vi "niFpgaRegisterEmulationRefIn.vi"(0 "Name":variant, 1 "in timed loop":bool, 7 "Data In":i32, 9 "Write? (F)":bool, 11 "error in (no error)":errorcluster, 12 "Node Link":cluster{"VIRef":refnum<vi>, "UID":i32}) -> (8 "Data Out":i32, 15 "error out":errorcluster)   [LabVIEW 2017]
uses:
  <vilib>/rvi/DataTransferAndStorage/Container/Common/niFpgaContainerMetaDataKey.ctl
  <instcachedir>/0/niFpgaRegisterEmulation_D83EC659CC8640A8A24FC76F9511FEDC.lvgen/niFpgaRegisterEmulation_D83EC659CC8640A8A24FC76F9511FEDC_000.vi
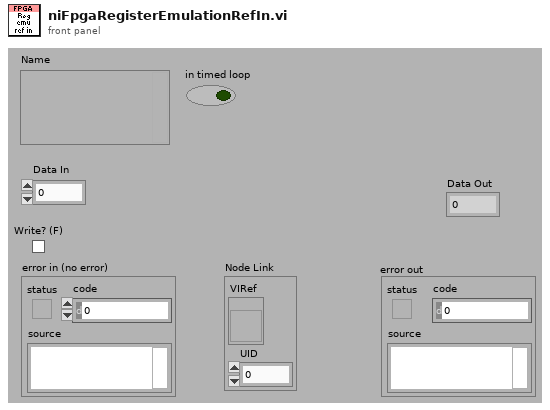
[diagram p1: front panel]
types:
  T1 = typedef "niFpgaContainerMetaDataKey.ctl" = enum16{"FPGA FIFO", "FPGA Memory", "FPGA Register", "FPGA Handshake"}
  T2 = typedef "niFpgaContainerState.ctl" = cluster{"displayName":string, "hardwareName":string, "dataType":T3, "elementTypeDescriptor":variant, "terminalTypeDescriptor":variant, "requestedNumberOfElements":u32, "memoryType":T4, "arbitrationForInterfaceA":T5, "numberOfElementsPerRead":u32, "arbitrationForInterfaceB":T5, "numberOfElementsPerWrite":u32, "VI_Defined":bool, "type":T6, "initializationParameters":T7, "disableOnOverflow/Underflow":bool, "interfaceConfiguration":T8, "controlLogic":T9, "actualNumberOfElements":u32, "dramSelection":string, "dramMaxOustandingRequests":i32, "dramIncludeByteEnables":bool, "dramGrantTime":u32, "fullEmulation":bool, "memoryInMultipleClockDomains":bool, "memoryLatency":T10}
  T3 = typedef "niFpgaDataTypeControl.ctl" = enum32{"Boolean", "I8", "I16", "I32", "I64", "U8", "U16", "U32", "U64", "FXP", "CustomControl", "SGL"}
  T4 = typedef "niFpgaContainerImplementationControl.ctl" = enum16{"Flip-Flops", "Look-Up Table", "Block Memory", "DRAM"}
  T5 = typedef "niFpgaContainerArbitrationOptionsControl.ctl" = enum16{"Always Arbitrate", "Arbitrate if Multiple Requestors Only", "Never Arbitrate"}
  T6 = typedef "niFpgaTransferTypeControl.ctl" = enum16{"Target-Scoped", "Host to Target - DMA", "Target to Host - DMA", "Peer to Peer Reader", "Peer to Peer Writer", "Bidirectional"}
  T7 = typedef "niFpgaContainerInitializationParameters.ctl" = cluster{"initialized":bool, "VI_Path":path, "initialData":variant}
  T8 = typedef "niFpgaMemoryInterfaceConfiguration.ctl" = enum16{"Read A-Write B", "Read A-Read B"}
  T9 = typedef "niFpgaFifoControlLogicControl.ctl" = enum16{"Slice Fabric", "Target Optimal", "Built-in"}
  T10 = typedef "niFpgaContainerMemoryLatencyControl.ctl" = u16
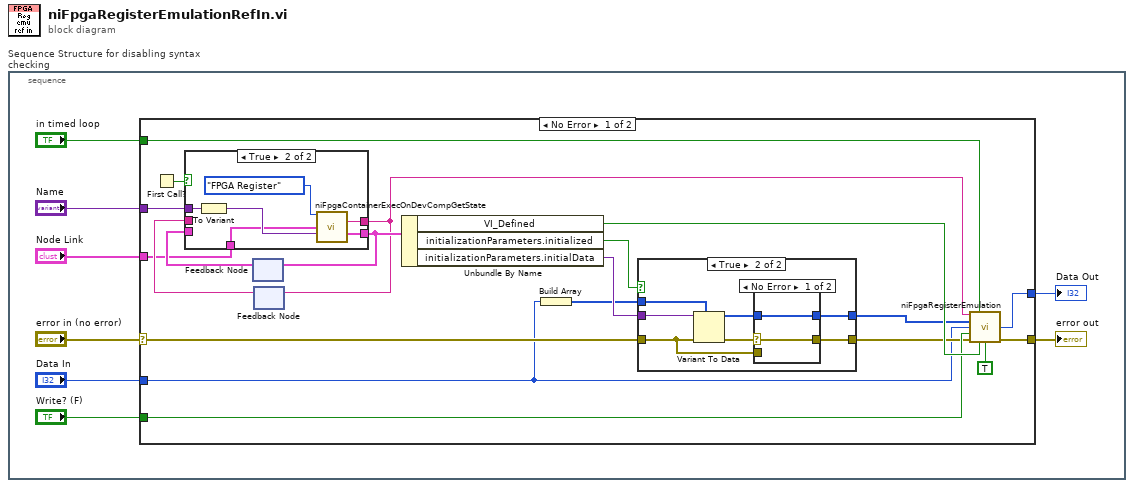
[diagram p0: block diagram]
diagram:
  n1 = stacked-sequence "Sequence Structure for disabling syntax checking" {
    frame #0 {
      n2 = case shown="No Error" "error in (no error)" {
        selector: "error in (no error)" -> [w23 w48]
        tunnel: [w17 w48] -> w1
        tunnel: "Name" -> [w27 _]
        tunnel: [w18 _] -> w2
        tunnel: "Data In" -> [w11 _]
        tunnel: "Write? (F)" -> [w19 _]
        tunnel: "in timed loop" -> [w14 _]
        tunnel: "Node Link" -> [w10 _]
        frame No Error {
          n3 = First Call?() -> (First Call?: T/F=w28:bool)
          n4 = feedback #1() -> (w25:T2)  [unwired: 1 out]
          n5 = feedback #2() -> (w24:string)  [unwired: 1 out]
          n6 = case shown="True" w28 {
            tunnel: w27 -> [_ w47]
            tunnel: [w41 w43] -> w26
            tunnel: w25 -> [w41 _]
            tunnel: [w40 w44] -> w21
            tunnel: w24 -> [w40 _]
            tunnel: w10 -> [_ w42]
            frame False {
            }
            frame True {
              n7 = To Variant(anything=w47) -> (Variant=w46:variant)
              n8 = call <vilib>:"niFpgaContainerExecOnDevCompGetState.vi"("containerMetaDataKey"=niFpgaContainerMetaDataKey."FPGA Register", "Node Link"=w42, "name"=w46) -> ("Unique  Name"=w44:string, "containerState"=w43:T2)  [unwired: 3 in, 8 out]
            }
          }
          n9 = feedback-in #1(w26) -> ()
          n10 = feedback-in #2(w21) -> ()
          n11 = Unbundle By Name(w26) -> ("VI_Defined"=w20:bool, "initializationParameters.initialized"=w15:bool, "initializationParameters.initialData"=w22:variant)
          n12 = Build Array(w11) -> (w12:i32[])
          n13 = case shown="True" w15 {
            tunnel: w23 -> [w29 w32]
            tunnel: w22 -> [_ w36]
            tunnel: [_ w30] -> w9
            tunnel: [w29 w33] -> w16
            tunnel: w12 -> [_ w35]
            frame False {
            }
            frame True {
              n14 = Variant To Data(error in=w32, type=w35, Variant=w36) -> (data=w31:i32[], error out=w34:errorcluster)
              n15 = case shown="No Error" w34 {
                selector: w34 -> [w38 _]
                tunnel: [w38 w39] -> w33
                tunnel: w32 -> [_ w39]
                tunnel: w31 -> [w37 _]
                tunnel: [w37 _] -> w30
                frame No Error {
                }
                frame Error {
                }
              }
            }
          }
          n16 = call-generic <vilib>:"niFpgaRegisterEmulation.vi"("name"=w21, "in timed loop"=w14, "Initial Value"=w9, "data in"=w11, "write"=w19, "error in (no error)"=w16, "Local? (F)"=w20, "Ref In wired (F)"=TRUE ("ref in wired")) -> ("data out"=w18:i32, "error out"=w17:errorcluster)  [unwired: 6 in]
        }
        frame Error {
        }
      }
      "error out" <- w1
      "Data Out" <- w2
    }
  }
